vi "Write Sub panel.vi"(10 "Sub panel":refnum<vi>, 11 "Si UI in":refnum<class "Si UI.lvclass">) -> (3 "Si UI out":refnum<class "Si UI.lvclass">)   [LabVIEW 2020, in "Si UI.lvlib" / "Si UI.lvclass"]
uses:
  Si UI.lvclass
  Si UI.lvclass/Si UI.ctl
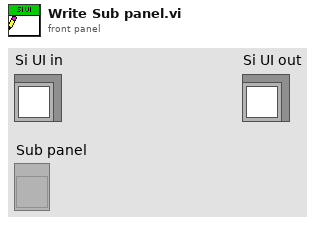
[diagram p1: front panel]
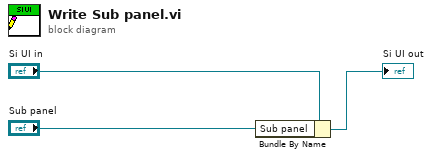
[diagram p0: block diagram]
diagram:
  n1 = Bundle By Name(cluster="Si UI in", "Sub panel"="Sub panel") -> (→"Si UI out":refnum<class "Si UI.lvclass">)
